vi "CAL-Show all.vi"(0 "Path":path, 5 "Mag graph":refnum<vi>, 7 "Phase graph":refnum<vi>, 11 "error in (no error)":errorcluster, 12 "Plot Max SPL":bool) -> (8 "speakers":string[](array[string]), 15 "error out":errorcluster)   [LabVIEW 2020]
doc: "This helper VI plots all of the in ear calibration files in the current experiment data folder.\n\nKEH 9/10/09"
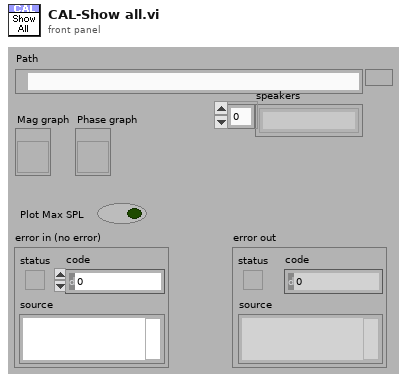
[diagram p1: front panel]
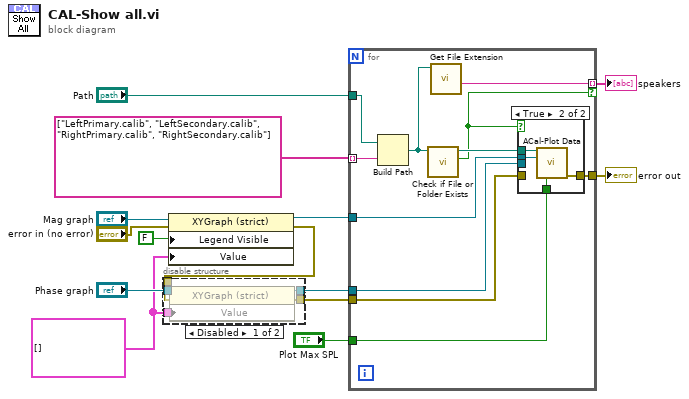
[diagram p0: block diagram]
diagram:
  w10 = cluster{"PTC Mag":dbl[], "PTC Phase":dbl[]}[] [] ("Value")
  n1 = property class="XYGraph (strict)"(reference="Mag graph", error in="error in (no error)", "Legend Visible"=FALSE ("Legend:Visible"), "Value"=w10) -> (reference out=w6:refnum<vi>, error out=w9:errorcluster)
  n2 = disable-structure shown="Disabled" {
    disable-tunnel: "Phase graph" -> [w19 _]
    disable-tunnel: w10 -> [w18 _]
    disable-tunnel: w9 -> [w17 _]
    disable-tunnel: [w16 _] -> w5
    disable-tunnel: [w15 _] -> w4
    frame Disabled {
      n3 = property class="XYGraph (strict)"(reference=w19, error in=w17, "Value"=w18) -> (reference out=w16:refnum<vi>, error out=w15:errorcluster)
    }
    frame Enabled {
    }
  }
  n4 = for {
    tunnel: string[] ["LeftPrimary.calib", "LeftSecondary.calib", "RightPrimary.calib", "RightSecondary.calib"] -> [w29] mode=indexing
    tunnel: "Path" -> [w30]
    tunnel: w6 -> [w28]
    tunnel: w5 -> [w27]
    tunnel: w4 -> [w26]
    tunnel: [w25] -> w3
    tunnel: "Plot Max SPL" -> [w23]
    tunnel: [w21] -> w1 mode=indexing if=w20
    n5 = Build Path(base path=w30, name or relative path=w29) -> (appended path=w22:path)
    n6 = call <vilib>:"Check if File or Folder Exists.vi"("path"=w22) -> ("file or folder exists?"=w20:bool, "dup path"=w24:path)  [unwired: 8 in, 1 out]
    n7 = call <vilib>:"Get File Extension.vi"("file"=w22) -> ("filename without extension"=w21:string)  [unwired: 6 in, 4 out]
    n8 = case shown="True" w20 {
      tunnel: w28 -> [_ w34]
      tunnel: w27 -> [_ _]
      tunnel: w26 -> [w31 _]
      tunnel: [w31 w33] -> w25
      tunnel: w24 -> [_ w35]
      tunnel: w23 -> [_ w32]
      frame False {
      }
      frame True {
        n9 = call "ACal-Plot Data.vi"("Path"=w35, "Mag graph"=w34, "Plot max"=w32) -> ("error out"=w33:errorcluster)  [unwired: 11 in, 1 out]
      }
    }
  }
  "error out" <- w3
  "speakers" <- w1
